vi "Create.vi"(7 "Sender":refnum<class "Sender.lvclass">, 9 "jettl":refnum<class "jettl.lvclass">, 10 "Self Alias":string, 11 "Base jettl in":refnum<class "Base jettl.lvclass">) -> (3 "Base jettl out":refnum<class "Base jettl.lvclass">)   [LabVIEW 2021, in "jettl.lvlib" / "Base jettl.lvclass"]
uses:
  Base jettl.lvclass
  Error/Error.lvlib
  Msg Strategy/Msg Strategy.lvclass
  Addresses Strategy/Addresses Strategy/Addresses Strategy.lvclass
  jettl/jettl.lvclass
  C:/git/jettl/jettl/jettl/jettl/jettl.lvclass
  C:/git/jettl/jettl/Create Msg Strategy/Create/Create.lvclass
  C:/git/jettl/jettl/jettl/Last Ack Creator Msg Strategy/Last Ack Creator/Last Ack Creator.lvclass
  C:/git/jettl/jettl/Merge Error Msg Strategy/Merge Error/Merge Error.lvclass
  C:/git/jettl/jettl/Override Error Msg Strategy/Override Error/Override Error.lvclass
  C:/git/jettl/jettl/Setup Msg Strategy/Setup/Setup.lvclass
  C:/git/jettl/jettl/Teardown Msg Strategy/Teardown/Teardown.lvclass
  Sender/Sender/Sender.lvclass
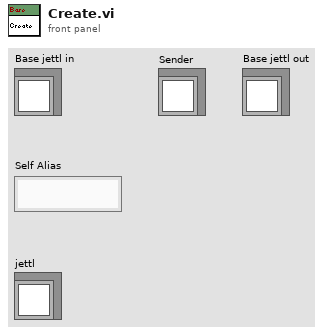
[diagram p1: front panel]
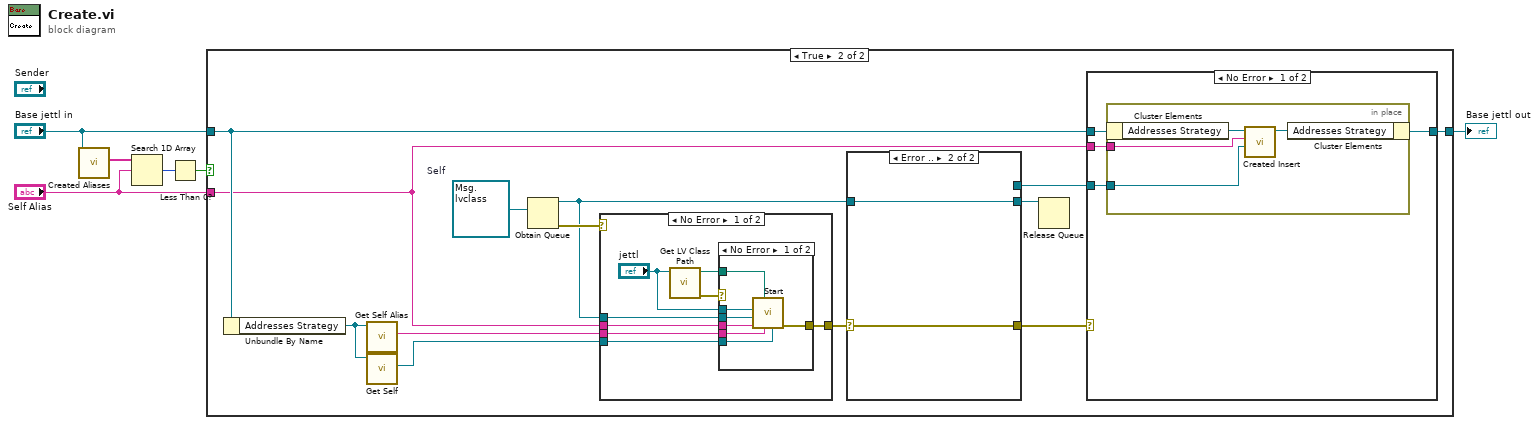
[diagram p0: block diagram]
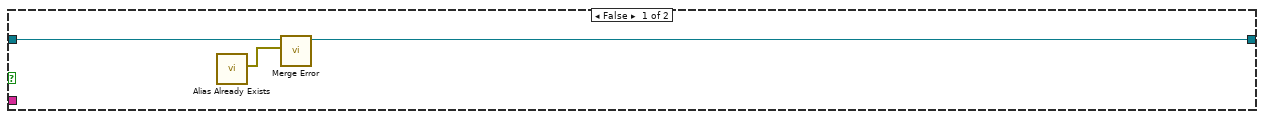
[diagram p2: hidden frame]
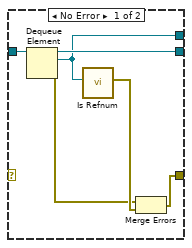
[diagram p3: hidden frame]
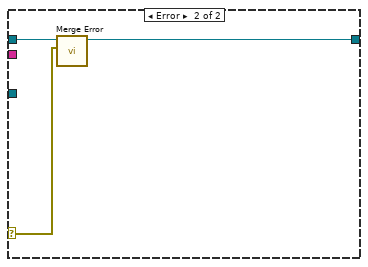
[diagram p6: hidden frame]
diagram:
  n1 = call-dynamic "Created Aliases.vi"("Base jettl in"="Base jettl in") -> ("Created Aliases"=w5:string[])  [unwired: 10 in]
  n2 = Search 1D Array(1D array=w5, element="Self Alias") -> (index of element=w3:i32)  [unwired: 1 in]
  n3 = Less Than 0?(x=w3) -> (x < 0?=w2:bool)
  n4 = case shown="True" w2 {
    tunnel: "Base jettl in" -> [w8 w17]
    tunnel: "Self Alias" -> [_ w11]
    tunnel: [w7 w22] -> w6
    frame False {
      n5 = call "Alias Already Exists.vi"() -> ("Error"=w9:errorcluster)  [unwired: 11 in]
      n6 = call-dynamic "Merge Error.vi"("Error"=w9, "Base jettl in"=w8) -> ("Base jettl out"=w7:refnum<class "Base jettl.lvclass">)  [unwired: 9 in]
    }
    frame True {
      w13 = refnum<user-event> refnum  # Self
      n7 = Unbundle By Name(w17) -> ("Addresses Strategy"=w16:refnum<class "Addresses Strategy.lvclass">)
      n8 = call-dynamic "Get Self Alias.vi"("Addresses Strategy in"=w16) -> ("Self Alias"=w14:string)  [unwired: 10 in]
      n9 = call-dynamic "Get Self.vi"("Addresses Strategy in"=w16) -> ("Self"=w15:refnum<user-event>)  [unwired: 10 in]
      n10 = Obtain Queue(element data type=w13) -> (queue out=w12:refnum<queue>, error out=w21:errorcluster)  [unwired: 4 in, 1 out]
      n11 = case shown="No Error" w21 {
        selector: w21 -> [_ w47]
        tunnel: [w38 w47] -> w19
        tunnel: w11 -> [w35 _]
        tunnel: w15 -> [w37 _]
        tunnel: w14 -> [w36 _]
        tunnel: w12 -> [w34 _]
        frame No Error {
          n12 = call <vilib>:"Get LV Class Path.vi"("object"="jettl") -> ("error out"=w31:errorcluster, "class path"=w32:path)  [unwired: 9 in]
          n13 = case shown="No Error" w31 {
            selector: w31 -> [_ w46]
            tunnel: [w45 w46] -> w38
            tunnel: w37 -> [w44 _]
            tunnel: w36 -> [w43 _]
            tunnel: w35 -> [w42 _]
            tunnel: w34 -> [w41 _]
            tunnel: "jettl" -> [w40 _]
            tunnel: w32 -> [w39 _]
            frame No Error {
              n14 = call "Start.vi"("Creator"=w44, "Creator Alias"=w43, "Path"=w39, "Self Alias"=w42, "Queue of Self"=w41, "jettl"=w40) -> ("error out"=w45:errorcluster)  [unwired: 5 in]
            }
            frame Error {
            }
          }
        }
        frame Error {
        }
      }
      n15 = case shown="Error .." w19 {
        selector: w19 -> [_ w30]
        tunnel: [w28 w30] -> w20
        tunnel: w12 -> [w26 w29]
        tunnel: [w23 _] -> w18
        tunnel: [w24 w29] -> w10
        frame No Error {
          n16 = Dequeue Element(queue=w26) -> (queue out=w24:refnum<queue>, element=w23:refnum<user-event>, error out=w25:errorcluster)  [unwired: 2 in, 1 out]
          n17 = call "Is Refnum.vi"("Self"=w23) -> ("Error"=w27:errorcluster)  [unwired: 10 in]
          n18 = Merge Errors(w25, w27) -> (w28:errorcluster)
        }
        frame Error {
        }
      }
      n19 = Release Queue(queue=w10) -> ()  [unwired: 2 in, 3 out]
      n20 = case shown="No Error" w20 {
        selector: w20 -> [_ w58]
        tunnel: w17 -> [w49 w57]
        tunnel: [w48 w56] -> w22
        tunnel: w18 -> [w51 _]
        tunnel: w11 -> [w50 _]
        frame No Error {
          n21 = in-place {
            in-place-border: w51 -> [w52]
            in-place-border: w50 -> [w53]
            n22 = in-place-cluster #1(w49) -> ("Addresses Strategy"=w55:refnum<class "Addresses Strategy.lvclass">)
            n23 = call-dynamic "Created Insert.vi"("Created"=w52, "Created Alias"=w53, "Addresses Strategy in"=w55) -> ("Addresses Strategy out"=w54:refnum<class "Addresses Strategy.lvclass">)  [unwired: 8 in]
            n24 = in-place-cluster #1("Addresses Strategy"=w54) -> (w48:refnum<class "Base jettl.lvclass">)
          }
        }
        frame Error {
          n25 = call-dynamic "Merge Error.vi"("Error"=w58, "Base jettl in"=w57) -> ("Base jettl out"=w56:refnum<class "Base jettl.lvclass">)  [unwired: 9 in]
        }
      }
    }
  }
  "Base jettl out" <- w6
